vi "IPs Array.vi"() -> (3 "IPs":refnum<class "Engine Simulation IP.lvclass">[](array[class]))   [LabVIEW 2013, in "Engine Simulation Session.lvclass"]
uses:
  Engine Simulation Session.lvclass
  Engine Simulation IP.lvclass
  Analog Replay/Analog Replay.lvclass
  APU/APU.lvclass
  Digital Pattern Generation/Digital Pattern Generation.lvclass
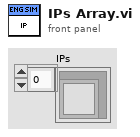
[diagram p1: front panel]
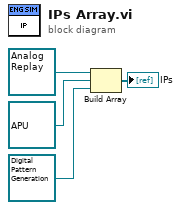
[diagram p0: block diagram]
diagram:
  n1 = Build Array(refnum<class "Analog Replay.lvclass"> refnum ("Analog Replay.lvclass"), refnum<class "APU.lvclass"> refnum ("APU.lvclass"), refnum<class "Digital Pattern Generation.lvclass"> refnum ("Digital Pattern Generation.lvclass")) -> (→"IPs":refnum<class "Engine Simulation IP.lvclass">[])
